vi "Insert  Result File Path to ResultsDB - Copy.vi"(6 "CMD":string(combo)="Insert", 7 "Save file OK":string, 8 "error in (no error)":errorcluster, 9 "appended path":path, 10 "StationName":string, 11 "Barcode":string) -> (0 "error out":errorcluster, 3 "Row Numbers":string)   [LabVIEW 2015]
doc: "保存测试结果文件到DB数据库。方便数据查询。"
uses:
  SQLite.lvclass
  <userlib>/LabSQL/LabSQL.lvlib
  <userlib>/sushu/sushu.lvlib
  vi.lib/TopPath.lvlib
panel:
  out "Select SQL CMD 3":string
  out "Table Control":string[][](table)
  out "Select SQL CMD 2":string
  out "match substring":string
  out "string":string
  out "Select SQL CMD":string
  out "number (0 to 1)":dbl
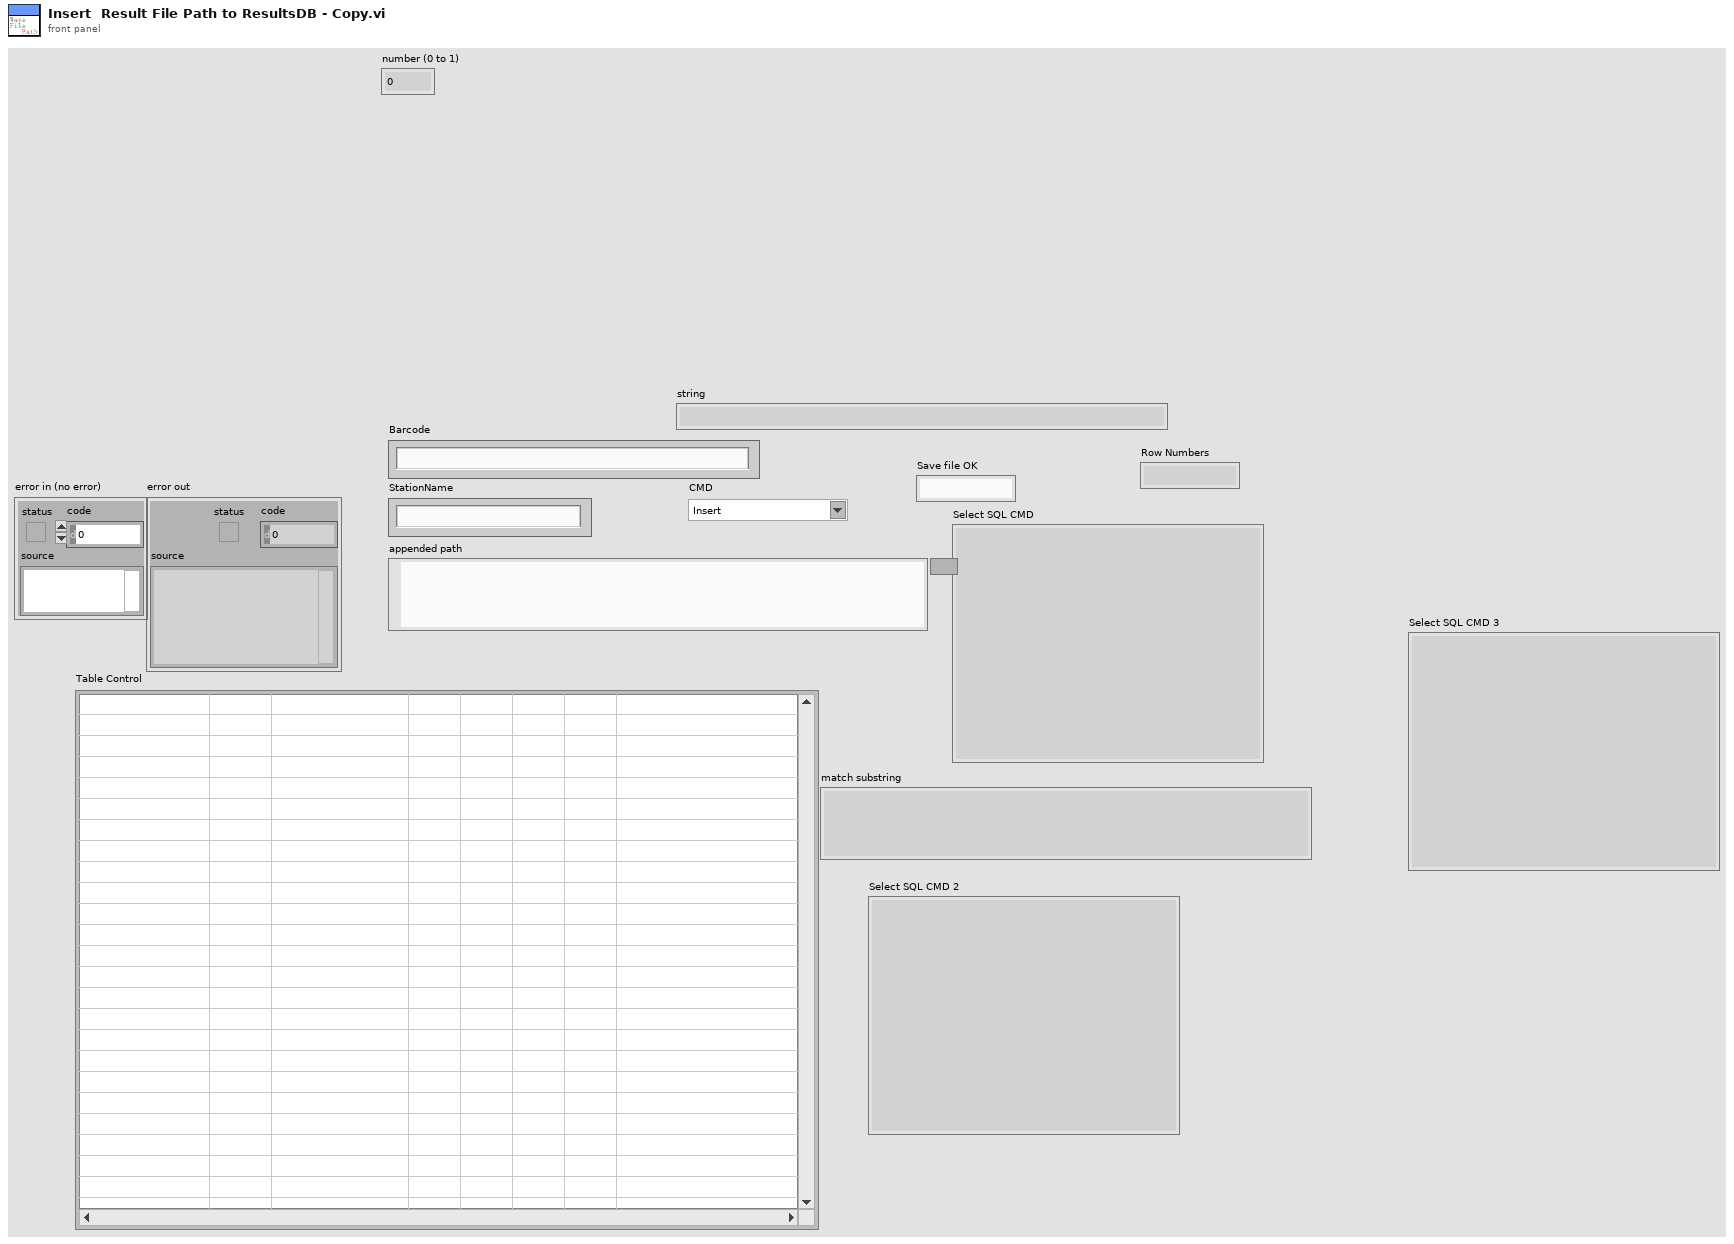
[diagram p1: front panel]
types:
  T1 = cluster{"Core":cluster{"Current VI Reference":refnum<vi>, "Close Panel on Exit?":bool}, "VI Name":string, "Row Numbers":string, "Update?":bool}
  T2 = typedef "sushu_vi_lib.lvlib/TopPath.lvlib/Top Path.ctl" = cluster{"LV Source":path, "FilePath":path, "Data":path}
  T3 = enum16{"Other", "SQL2008", "SQLite", "Access", "MySQL"}
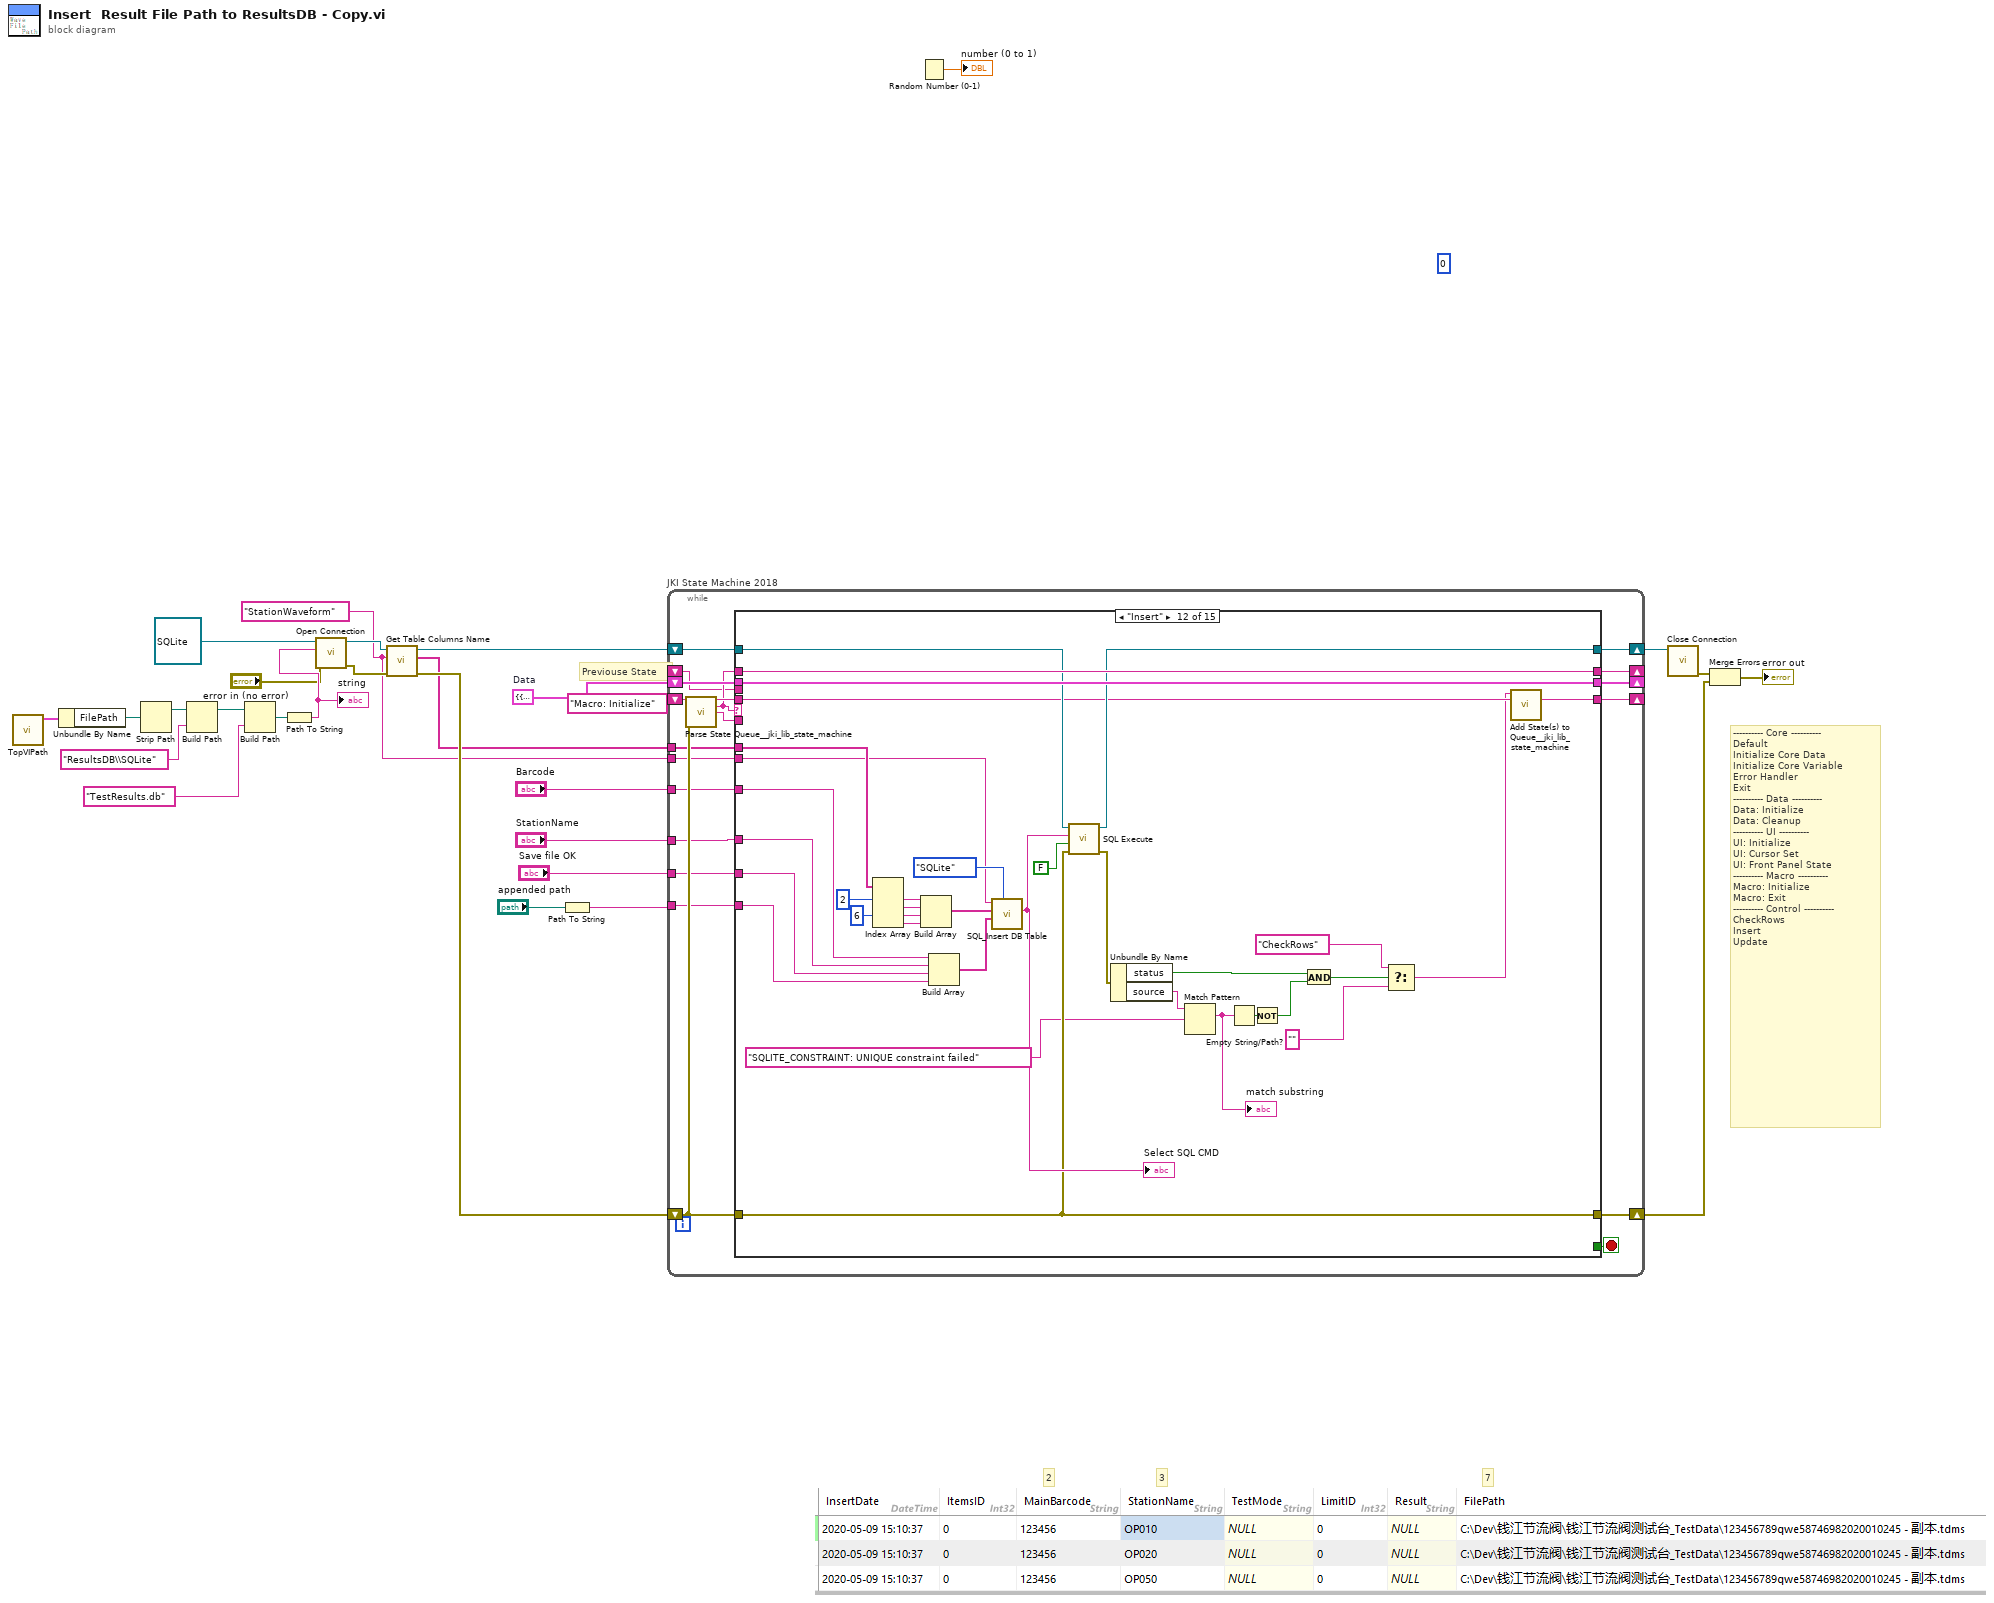
[diagram p0: block diagram]
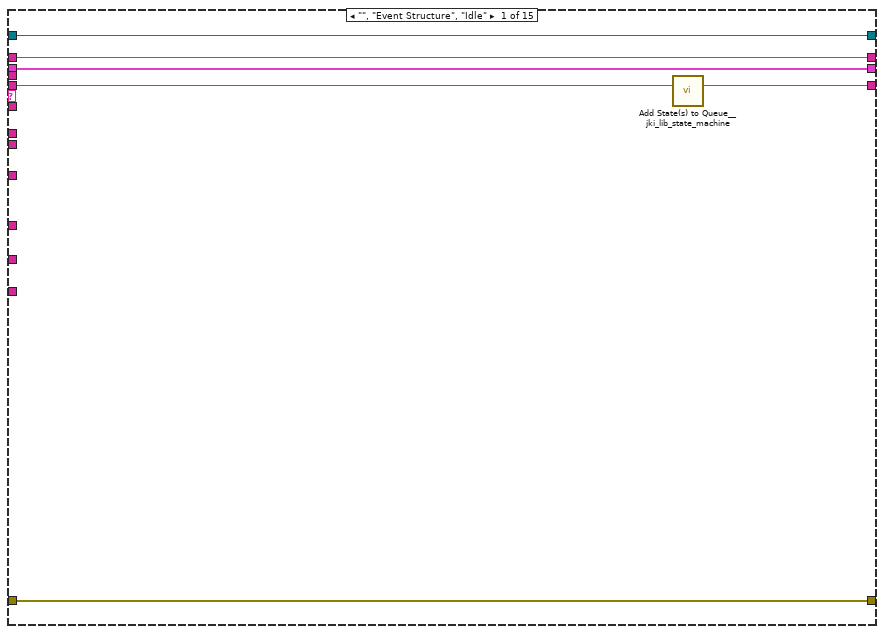
[diagram p2: hidden frame]
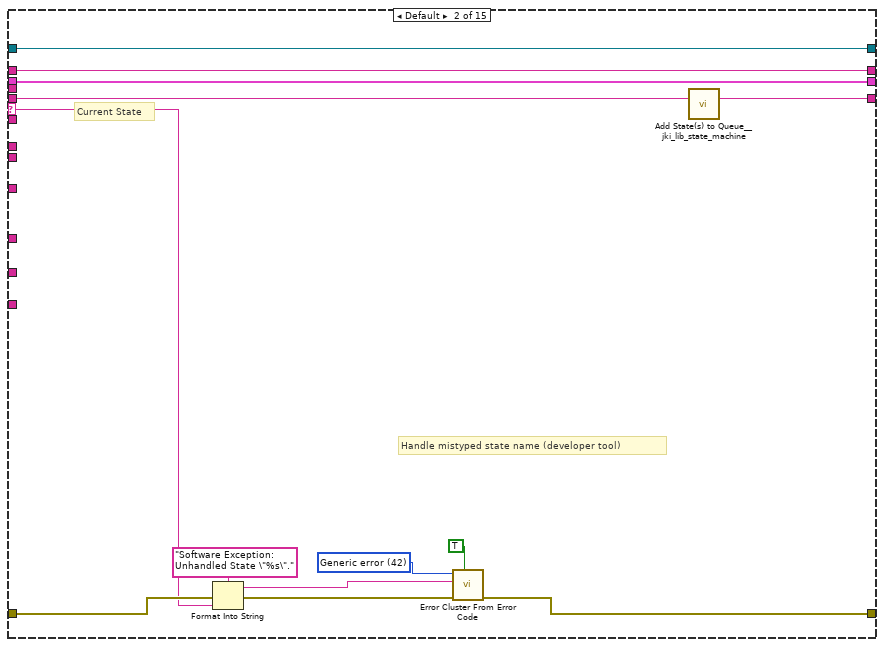
[diagram p3: hidden frame]
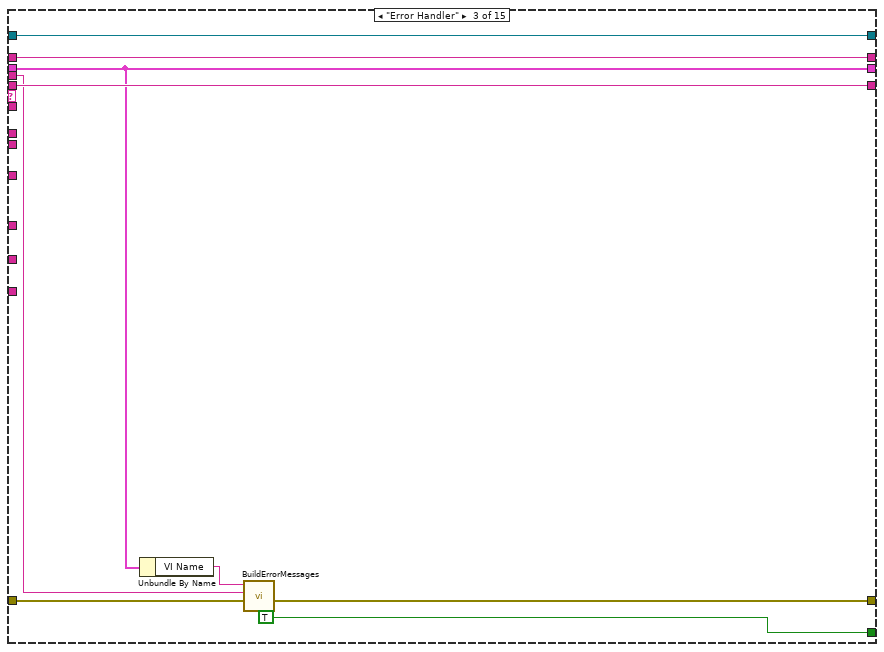
[diagram p4: hidden frame]
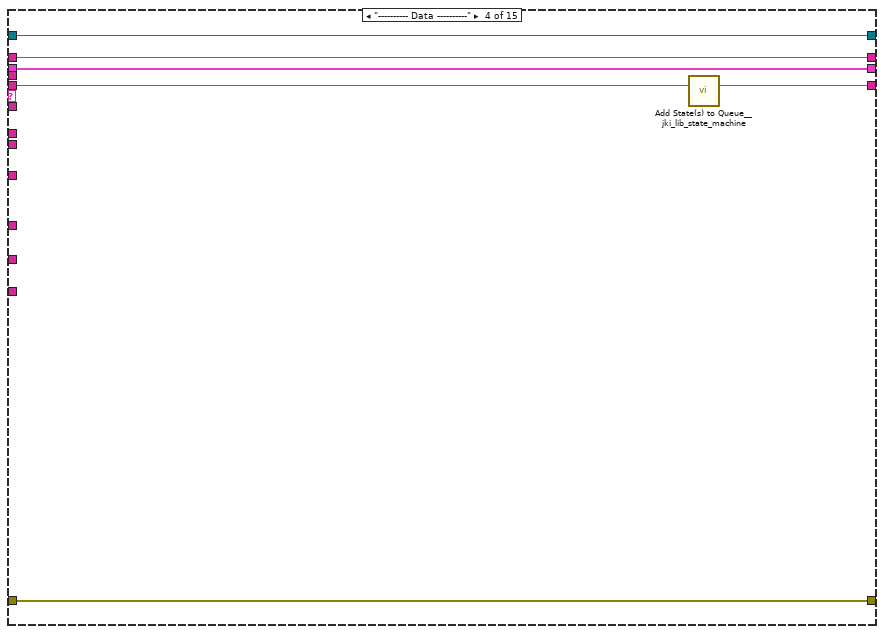
[diagram p5: hidden frame]
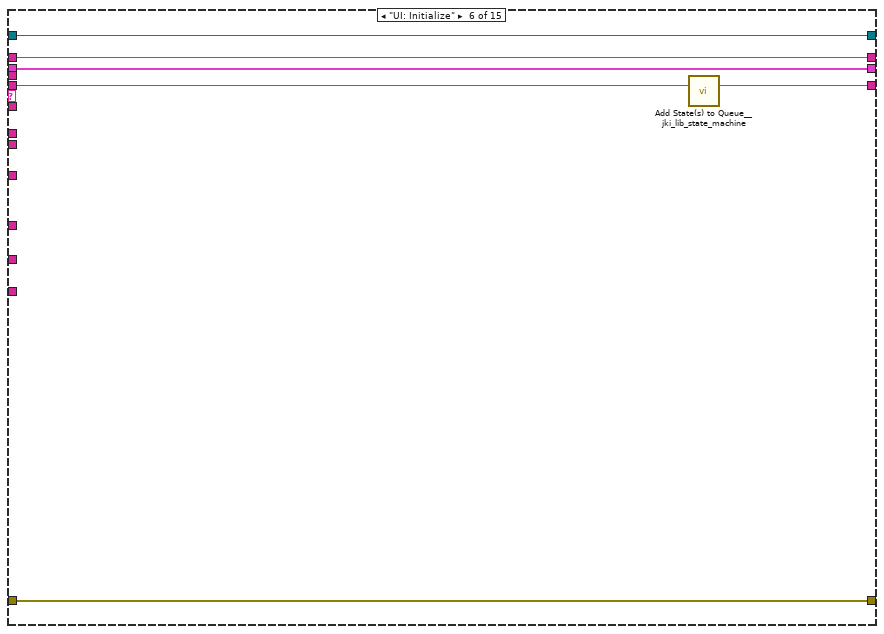
[diagram p7: hidden frame]
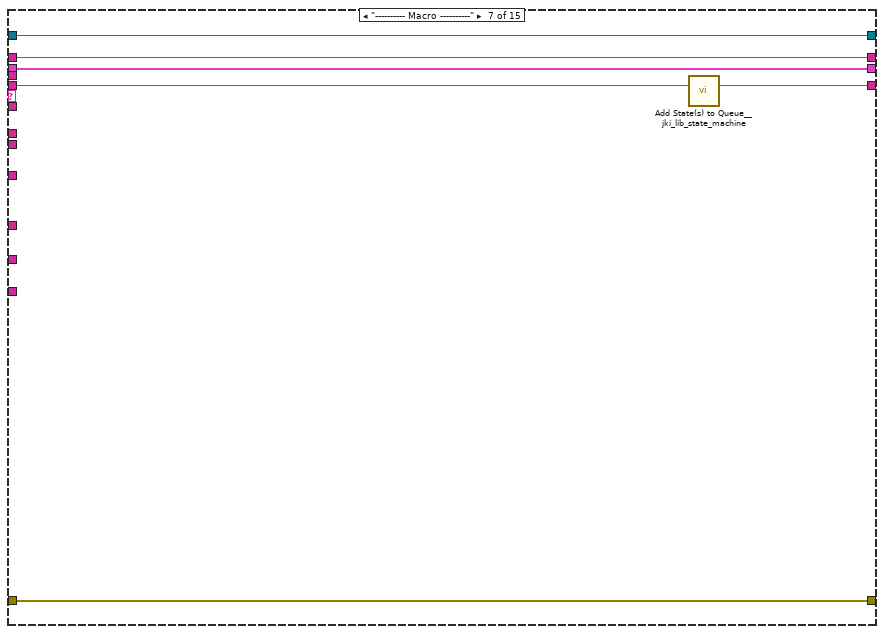
[diagram p8: hidden frame]
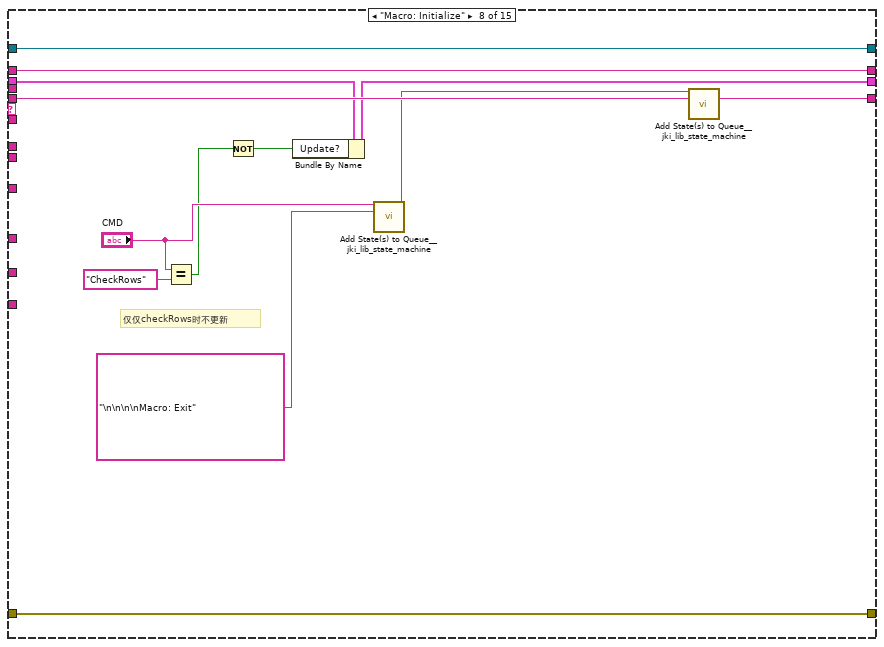
[diagram p9: hidden frame]
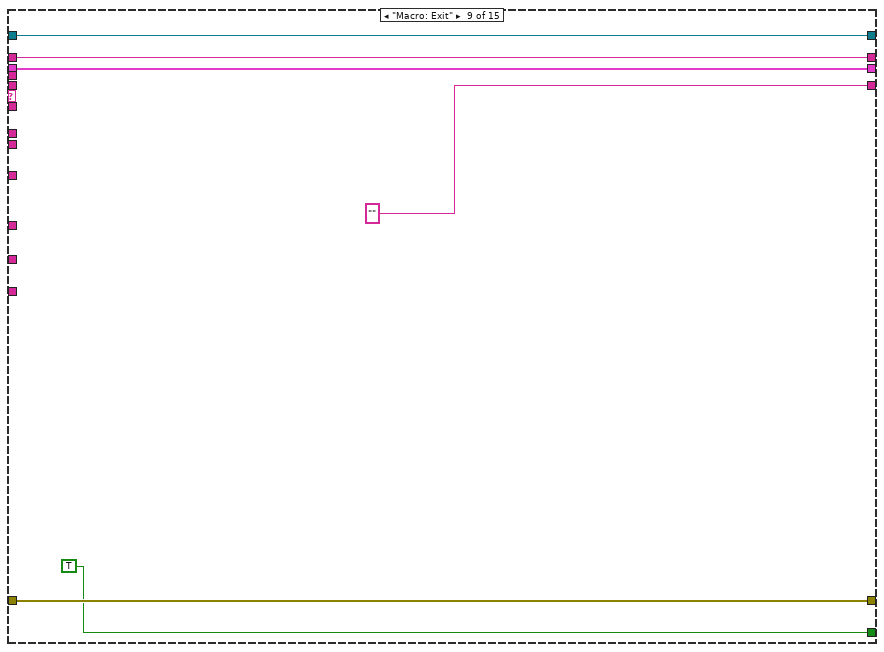
[diagram p10: hidden frame]
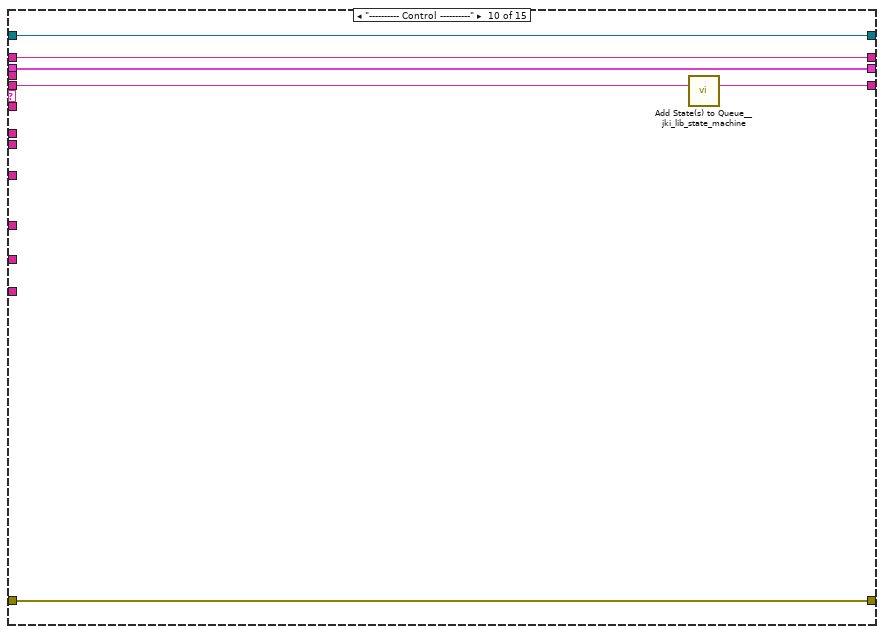
[diagram p11: hidden frame]
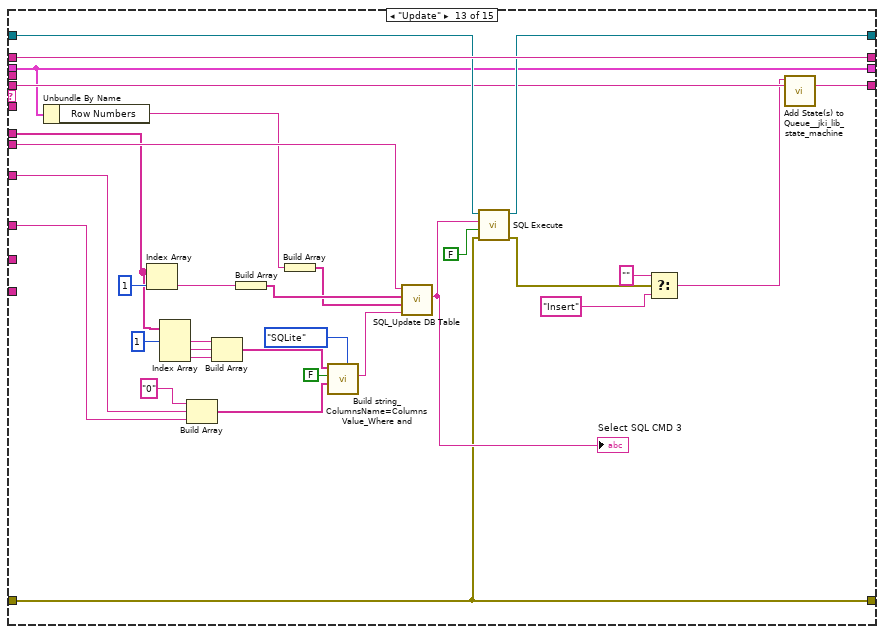
[diagram p13: hidden frame]
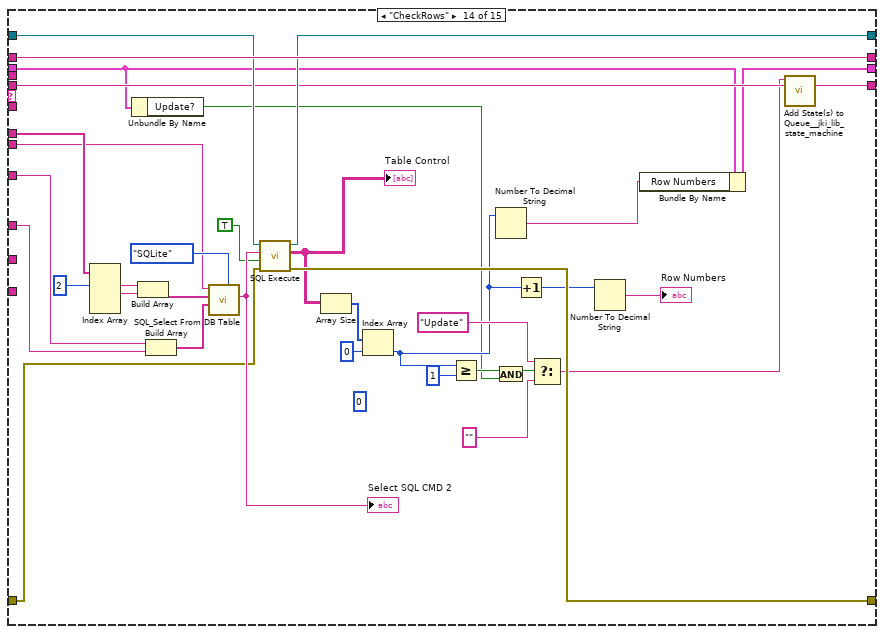
[diagram p14: hidden frame]
diagram:
  w12 = T1 {"Core"={"Current VI Reference"=refnum, "Close Panel on Exit?"=FALSE}, "VI Name"="", "Row Numbers"="", "Update?"=FALSE}  # Data
  (unwired) 0 ("index (row)")
  w1 = "StationWaveform" ("TableName")
  # "Previouse State"
  # "---------- Core ----------\nDefault\nInitialize Core Data\nInitialize Core Variable\nError Handler\nExit\n---------- Data ----------\nData: Initialize\nData: Cleanup\n---------- UI ----------\nUI: Initialize\nUI: Cursor Set\nUI: Front Panel State\n---------- Macro ----------\nMacro: Initialize\nMacro: Exit\n---------- Control ----------\nCheckRows\nInsert\nUpdate"
  # "7"
  # "3"
  # "2"
  n1 = call "TopVIPath.vi"() -> ("TopPath"=w14:T2)  [unwired: 10 in, 1 out]
  n2 = Unbundle By Name(w14) -> ("FilePath"=w27:path)
  n3 = Strip Path(path=w27) -> (stripped path=w26:path)  [unwired: 1 out]
  n4 = Build Path(base path=w26, name or relative path="ResultsDB\\SQLite") -> (appended path=w24:path)
  n5 = Build Path(base path=w24, name or relative path="TestResults.db") -> (appended path=w22:path)
  n6 = Path To String(path=w22) -> (string=w21:string)
  "string" <- w21
  n7 = call-dynamic "Open Connection.vi"("error in (no error)"="error in (no error)", "ConnectionString"=w21, "HostDB in"=refnum<class "SQLite.lvclass"> refnum ("SQLite.lvclass")) -> ("error out"=w18:errorcluster, "HostDB out"=w19:refnum<class "SQLite.lvclass">)  [unwired: 7 in]
  n8 = call-dynamic "Get Table Columns Name.vi"("error in (no error)"=w18, "TableName"=w1, "HostDB in"=w19) -> ("error out"=w7:errorcluster, "ColunmsList"=w2:string[], "HostDB out"=w11:refnum<class "SQLite.lvclass">)  [unwired: 4 in, 2 out]
  n9 = Path To String(path="appended path") -> (string=w6:string)
  n10 = while "JKI State Machine 2018" {
    shift-right: [w42] -> _
    shift-left: w12 -> [w41]
    shift-right: [w45] -> w8
    shift-left: w7 -> [w40]
    shift-right: [w44] -> _
    shift-left: "Macro: Initialize" -> [w46]
    shift-right: [w38] -> w10
    shift-left: w11 -> [w39]
    shift-right: [w36] -> _
    shift-left: _ -> [w35]
    tunnel: w6 -> [w34]
    tunnel: "Save file OK" -> [w33]
    tunnel: "StationName" -> [w32]
    tunnel: "Barcode" -> [w31]
    tunnel: w2 -> [w30]
    tunnel: w1 -> [w29]
    stop <- w43 stop-if-true
    n11 = call <vilib>:"Parse State Queue__jki_lib_state_machine.vi"("State Queue"=w46, "Error In (no error)"=w40) -> ("Remaining States"=w48:string, "Current State"=w37:string, "Arguments"=w47:string)  [unwired: 11 in]
    n12 = case shown="\"Insert\"" w37 {
      selector: w37 -> [_ w57 _ _ _ _ _ _ _ _ _ _ _ _ _]
      tunnel: w48 -> [w54 w61 w75 w82 w84 w93 w99 w112 _ w124 w129 w132 w183 w215 w235]
      tunnel: w47 -> [_ _ _ _ _ _ _ _ _ _ _ _ _ _ _]
      tunnel: w41 -> [w51 w59 w72 w79 w85 w91 w96 w107 w117 w121 w128 w164 w182 w199 w234]
      tunnel: [w52 w63 w68 w80 w87 w90 w97 w108 w118 w122 w125 w143 w185 w213 w236] -> w45
      tunnel: w40 -> [w52 w62 w69 w80 w87 w90 w97 w108 w118 w122 w125 w143 w185 w214 w236]
      tunnel: [w53 w60 w75 w81 w84 w92 w98 w111 "" w123 w129 w133 w184 w216 w235] -> w44
      tunnel: [_ _ TRUE _ _ _ _ _ TRUE _ _ _ _ _ _] -> w43
      tunnel: [w51 w59 w72 w79 w85 w91 w96 w102 w117 w121 w128 w164 w182 w204 w234] -> w42
      tunnel: w39 -> [w50 w56 w74 w78 w86 w89 w95 w110 w116 w120 w127 w147 w189 w220 w233]
      tunnel: [w50 w56 w74 w78 w86 w89 w95 w110 w116 w120 w127 w146 w188 w219 w233] -> w38
      tunnel: w37 -> [w49 w55 w73 w77 w83 w88 w94 w109 w114 w119 w126 w163 w196 w231 w232]
      tunnel: [w49 w55 w73 w77 w83 w88 w94 w109 w114 w119 w126 w163 w196 w231 w232] -> w36
      tunnel: w35 -> [_ _ w70 _ _ _ _ _ _ _ _ _ _ _ _]
      tunnel: w34 -> [_ _ _ _ _ _ _ _ _ _ _ w148 _ _ _]
      tunnel: w33 -> [_ _ _ _ _ _ _ _ _ _ _ w149 _ _ _]
      tunnel: w32 -> [_ _ _ _ _ _ _ _ _ _ _ w150 w190 w221 _]
      tunnel: w31 -> [_ _ _ _ _ _ _ _ _ _ _ w151 w191 w222 _]
      tunnel: w30 -> [_ _ _ _ _ _ _ _ _ _ _ w153 w177 w224 _]
      tunnel: w29 -> [_ _ _ _ _ _ _ _ _ _ _ w152 w192 w223 _]
      frame "", "Event Structure", "Idle" {
        n13 = call <vilib>:"Add State(s) to Queue__jki_lib_state_machine.vi"("State(s) in (\"\")"=w54) -> ("States Out"=w53:string)  [unwired: 14 in]
      }
      frame Default {
        w66 = 42 items=["No error", "Argument error", "Memory is full", "Out of zone", "End of file", "File already open", "Generic file I/O error", "File not found", "File permission error", "Disk is full", "Duplicate path", "Too many files open", "System feature not enabled", "Resource file not found", "Cannot add resource", "Resource not found", "Image not found", "Image memory error", "Pen does not exist", "Config type invalid", "Config token not found", "Config parse error", "Config memory error", "Bad external code format", "Bad external code offset", "External code not present", "Null window", "Destroy window error", "Null menu", "Print aborted", "Bad print record", "Print driver error", "Windows error during printing", "Memory error during printing", "Print dialog error", "Generic print error", "Invalid device refnum", "Device not found", "Device parameter error", "Device unit error", "Cannot open device", "Device call aborted", "Generic error", "Cancelled by user", "Object ID too low", "Object ID too high", "Object not in heap", "Unknown heap", "Unknown object (invalid DefProc)", "Unknown object (DefProc not in table)", "Message out of range", "Invalid (null) method", "Unknown message", "Manager call not supported", "Bad address", "Network operation in progress", "Network operation timed out", "Connection is busy", "Network attribute not supported", "Network error", "Address in use", "System out of memory", "Connection aborted", "Connection refused", "Not connected", "Already connected", "Connection closed", "Initialization error (interapplication manager)", "Bad occurrence", "Wait on unbound occurrence handler", "Occurrence queue overflow", "Datalog type conflict", "Unused", "Unrecognized type (interapplication manager)", "Memory corrupt", "Failed to make temporary DLL", "Old CIN version", "Drag socket not found", "Failed to load drop-object", "Failed to register OLE object", "Failed to release OLE object", "Format specifier type mismatch", "Unknown format specifier", "Too few format specifiers", "Too many format specifiers", "Scan failed", "Newer CIN version", "Error converting to variant", "Runtime menu error", "Password tampered", "Variant attribute not found", "Incompatible variant data type", "Event data is not available", "Event Store is not present", "Occurrence is not found", "Event Queue is not created", "Event info is not available", "Refnum passed is NULL", "Error retrieving Class GUID", "Error retrieving CoClass GUID", "Error retrieving TypeLib GUID.", "Bad built application magic bytes.", "Specific driver is different from the specific driver associated with the Logical Name.", "There is no session opened to the class driver.", "Max Error", "MAX - Error with config objects", "MAX - Error loading configuration", "MAX - Group not supported"]
        # "Current State"
        # "Handle mistyped state name (developer tool)"
        n14 = Format Into String(format string="Software Exception: Unhandled State \"%s\"." ("message"), error in=w62, w57) -> (resulting string=w65:string, error out=w64:errorcluster)  [unwired: 1 in]
        n15 = call <vilib>:"Error Cluster From Error Code.vi"("show call chain? (False)"=TRUE, "error in (no error)"=w64, "error message (\"\")"=w65, "error code (0)"=w66) -> ("error out"=w63:errorcluster)  [unwired: 5 in]
        n16 = call <vilib>:"Add State(s) to Queue__jki_lib_state_machine.vi"("State(s) in (\"\")"=w61) -> ("States Out"=w60:string)  [unwired: 14 in]
      }
      frame "Error Handler" {
        n17 = Unbundle By Name(w72) -> ("VI Name"=w71:string)
        n18 = call <userlib>:"BuildErrorMessages.vi"("error in"=w69, "ErrorCase"=w70, "VI Name"=w71) -> ("error out (no error)"=w68:errorcluster)  [unwired: 6 in, 2 out]
      }
      frame "---------- Data ----------" {
        n19 = call <vilib>:"Add State(s) to Queue__jki_lib_state_machine.vi"("State(s) in (\"\")"=w82) -> ("States Out"=w81:string)  [unwired: 14 in]
      }
      frame "Data: Initialize" {
      }
      frame "UI: Initialize" {
        n20 = call <vilib>:"Add State(s) to Queue__jki_lib_state_machine.vi"("State(s) in (\"\")"=w93) -> ("States Out"=w92:string)  [unwired: 14 in]
      }
      frame "---------- Macro ----------" {
        n21 = call <vilib>:"Add State(s) to Queue__jki_lib_state_machine.vi"("State(s) in (\"\")"=w99) -> ("States Out"=w98:string)  [unwired: 14 in]
      }
      frame "Macro: Initialize" {
        # "仅仅checkRows时不更新"
        n22 = Equal?(x="CMD", y="CheckRows") -> (x = y?=w101:bool)
        n23 = Not(x=w101) -> (.not. x?=w100:bool)
        n24 = Bundle By Name(cluster=w107, "Update?"=w100) -> (w102:T1)
        n25 = call <vilib>:"Add State(s) to Queue__jki_lib_state_machine.vi"("State(s) in Front (\"\")"="CMD", "State(s) in (\"\")"="\n\n\n\nMacro: Exit") -> ("States Out"=w106:string)  [unwired: 13 in]
        n26 = call <vilib>:"Add State(s) to Queue__jki_lib_state_machine.vi"("State(s) in Front (\"\")"=w106, "State(s) in (\"\")"=w112) -> ("States Out"=w111:string)  [unwired: 13 in]
      }
      frame "Macro: Exit" {
      }
      frame "---------- Control ----------" {
        n27 = call <vilib>:"Add State(s) to Queue__jki_lib_state_machine.vi"("State(s) in (\"\")"=w124) -> ("States Out"=w123:string)  [unwired: 14 in]
      }
      frame "State1" {
      }
      frame "Insert" {
        n28 = Index Array(array=w153, index #1=2 ("index"), index #3=6 ("index")) -> (element #1=w158:string, element #2=w159:string, element #3=w160:string, element #4=w161:string)  [unwired: 2 in]
        n29 = Build Array(w158, w159, w160, w161) -> (w156:string[])
        n30 = Build Array(w151, w150, w149, w148) -> (w155:string[])
        n31 = call <userlib>:"SQL_Insert DB Table.vi"("DB Type"=T3."SQLite", "ColumnsValue"=w155, "ColumnsName"=w156, "Table Name"=w152) -> ("Insert DB String"=w145:string)  [unwired: 7 in]
        "Select SQL CMD" <- w145
        n32 = call-dynamic "SQL Execute.vi"("error in (no error)"=w143, "Return Data (T)"=FALSE, "Command Text"=w145, "HostDB in"=w147) -> ("error out"=w142:errorcluster, "HostDB out"=w146:refnum<class "SQLite.lvclass">)  [unwired: 3 in, 3 out]
        n33 = Unbundle By Name(w142) -> ("status"=w138:bool, "source"=w141:string)
        n34 = Match Pattern(string=w141, regular expression="SQLITE_CONSTRAINT: UNIQUE constraint failed") -> (match substring=w139:string)  [unwired: 1 in, 3 out]
        "match substring" <- w139
        n35 = Empty String/Path?(string/path=w139) -> (empty?=w137:bool)
        n36 = Not(x=w137) -> (.not. x?=w130:bool)
        n37 = And(x=w138, y=w130) -> (x .and. y?=w136:bool)
        n38 = Select(t="CheckRows", s=w136, f="") -> (s? t:f=w131:string)
        n39 = call <vilib>:"Add State(s) to Queue__jki_lib_state_machine.vi"("State(s) in Front (\"\")"=w131, "State(s) in (\"\")"=w132) -> ("States Out"=w133:string)  [unwired: 13 in]
      }
      frame "Update" {
        n40 = Unbundle By Name(w182) -> ("Row Numbers"=w181:string)
        n41 = Index Array(array=w177, index=1) -> (element=w195:string)
        n42 = Index Array(array=w177, index #1=1 ("index")) -> (element #1=w176:string, element #2=w175:string, element #3=w174:string)  [unwired: 2 in]
        n43 = Build Array("0" ("element"), w191, w190) -> (w171:string[])
        n44 = Build Array(w176, w175, w174) -> (w173:string[])
        n45 = Build Array(w195) -> (w193:string[])
        n46 = Build Array(w181) -> (w180:string[])
        n47 = call <userlib>:"Build string_ColumnsName=ColumnsValue_Where and.vi"("DB Type"=T3."SQLite", "ColumnsValue"=w171, "Check ASCII?"=FALSE, "ColumnsNameList"=w173) -> ("ColumnName='ColumnValue'"=w179:string)  [unwired: 7 in]
        n48 = call <userlib>:"SQL_Update DB Table.vi"("where name='value'"=w179, "ColumnsValue"=w180, "ColumnsNameList"=w193, "TableName"=w192) -> ("Update CMD"=w187:string)  [unwired: 7 in]
        "Select SQL CMD 3" <- w187
        n49 = call-dynamic "SQL Execute.vi"("error in (no error)"=w185, "Return Data (T)"=FALSE, "Command Text"=w187, "HostDB in"=w189) -> ("error out"=w168:errorcluster, "HostDB out"=w188:refnum<class "SQLite.lvclass">)  [unwired: 3 in, 3 out]
        n50 = Select(t="", s=w168, f="Insert") -> (s? t:f=w166:string)
        n51 = call <vilib>:"Add State(s) to Queue__jki_lib_state_machine.vi"("State(s) in Front (\"\")"=w166, "State(s) in (\"\")"=w183) -> ("States Out"=w184:string)  [unwired: 13 in]
      }
      frame "CheckRows" {
        (unwired) 0 ("element")
        n52 = Index Array(array=w224, index #1=2 ("index")) -> (element #1=w229:string, element #2=w230:string)  [unwired: 3 in, 2 out]
        n53 = Unbundle By Name(w199) -> ("Update?"=w197:bool)
        n54 = Build Array(w229, w230) -> (w227:string[])
        n55 = Build Array(w222, w221) -> (w226:string[])
        n56 = call <userlib>:"SQL_Select From DB Table.vi"("DB Type"=T3."SQLite", "ColumnsValue"=w226, "ColumnsNameList"=w227, "TableName"=w223) -> ("Select SQL CMD"=w218:string)  [unwired: 7 in]
        "Select SQL CMD 2" <- w218
        n57 = call-dynamic "SQL Execute.vi"("error in (no error)"=w214, "Return Data (T)"=TRUE, "Command Text"=w218, "HostDB in"=w220) -> ("error out"=w213:errorcluster, "Table Control"=w212:string[][], "HostDB out"=w219:refnum<class "SQLite.lvclass">)  [unwired: 3 in, 2 out]
        "Table Control" <- w212
        n58 = Array Size(array=w212) -> (size(s)=w211:i32[])
        n59 = Index Array(array=w211, index=0) -> (element=w203:i32)
        n60 = Greater Or Equal?(x=w203, y=1) -> (x >= y?=w208:bool)
        n61 = Number To Decimal String(number=w203) -> (decimal integer string=w201:string)  [unwired: 1 in]
        n62 = And(x=w208, y=w197) -> (x .and. y?=w198:bool)
        n63 = Increment(x=w203) -> (x+1=w202:i32)
        n64 = Select(t="Update", s=w198, f="") -> (s? t:f=w206:string)
        n65 = Number To Decimal String(number=w202) -> (decimal integer string=→"Row Numbers":string)  [unwired: 1 in]
        n66 = Bundle By Name(cluster=w199, "Row Numbers"=w201) -> (w204:T1)
        n67 = call <vilib>:"Add State(s) to Queue__jki_lib_state_machine.vi"("State(s) in Front (\"\")"=w206, "State(s) in (\"\")"=w215) -> ("States Out"=w216:string)  [unwired: 13 in]
      }
      frame "State3" {
      }
    }
  }
  n68 = Random Number (0-1)() -> (number: 0 to 1=→"number (0 to 1)":dbl)
  n69 = call-dynamic "Close Connection.vi"("HostDB in"=w10) -> ("error out"=w17:errorcluster)  [unwired: 9 in, 1 out]
  n70 = Merge Errors(w17, w8) -> (→"error out":errorcluster)
